vi "Verzoegerung.vi"(7 "Abfallverzögerung?":bool, 8 "ms":u16, 9 "sec":u16, 10 "min":u16, 11 "Startsignal":bool) -> (0 "Aktuelle Zeit [sec]":sgl, 3 "Zeit abgelaufen?":bool)   [LabVIEW 2020, in "Allgemein.lvlib"]
uses:
  Allgemein.lvlib
panel:
  # "VI Einstellung:\nAblaufinvarinate Ausführung\nKopie für jede Instanz vorbelegen\n(behält Zustand für jede Instanz bei)"
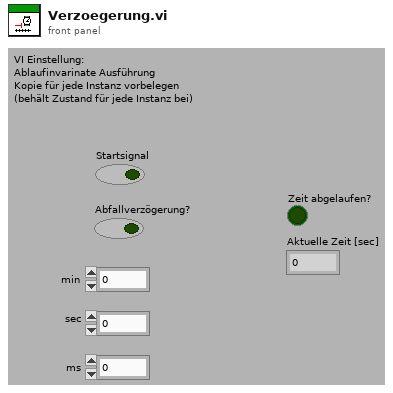
[diagram p1: front panel]
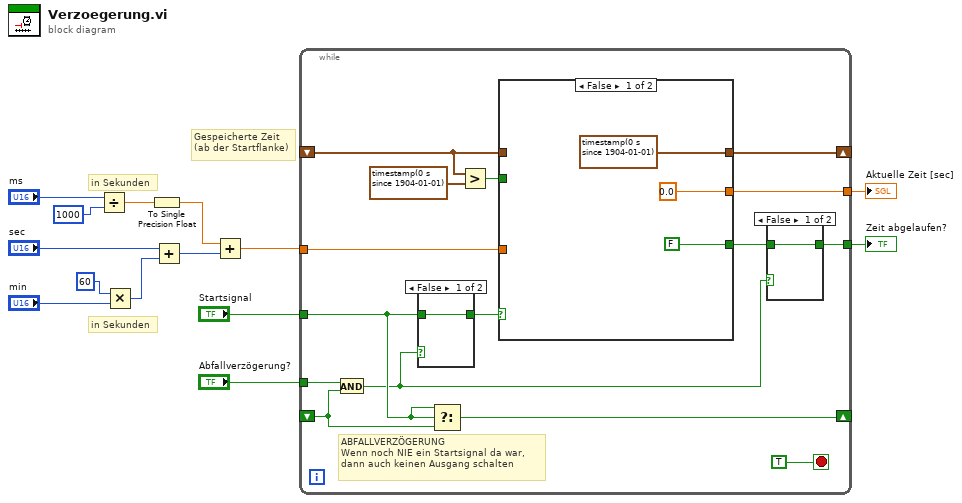
[diagram p0: block diagram]
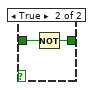
[diagram p2: hidden frame]
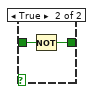
[diagram p3: hidden frame]
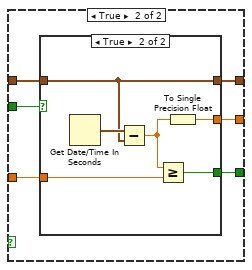
[diagram p4: hidden frame]
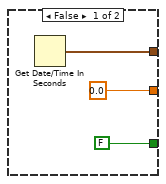
[diagram p5: hidden frame]
diagram:
  # "in Sekunden"
  # "in Sekunden"
  # "Gespeicherte Zeit\n(ab der Startflanke)"
  n1 = Divide(x="ms", y=u16 1000) -> (x/y=w3:dbl)
  n2 = Multiply(x=u16 60 ("y"), y="min") -> (x*y=w10:u16)
  n3 = To Single Precision Float(number=w3) -> (single precision float=w2:sgl)
  n4 = Add(x="sec", y=w10) -> (x+y=w6:u16)
  n5 = Add(x=w2, y=w6) -> (x+y=w5:sgl)
  n6 = while {
    shift-right: [w28] -> _
    shift-left: _ -> [w27]
    tunnel: w5 -> [w25]
    tunnel: "Startsignal" -> [w19]
    tunnel: [w24] -> w13
    tunnel: "Abfallverzögerung?" -> [w17]
    tunnel: [w20] -> w1
    shift-right: [w18] -> _
    shift-left: _ -> [w16]
    stop <- TRUE stop-if-true
    # "ABFALLVERZÖGERUNG\nWenn noch NIE ein Startsignal da war, \ndann auch keinen Ausgang schalten"
    n7 = And(x=w17, y=w16) -> (x .and. y?=w15:bool)
    n8 = case shown="False" w15 {
      tunnel: w19 -> [w33 w35]
      tunnel: [w33 w34] -> w21
      frame False {
      }
      frame True {
        n9 = Not(x=w35) -> (.not. x?=w34:bool)
      }
    }
    n10 = Select(t=w19, s=w19, f=w16) -> (s? t:f=w18:bool)
    n11 = Greater?(x=w27, y=timestamp(0 s since 1904-01-01) ("Aktuelle Zeit")) -> (0:w26:bool)
    n12 = case shown="False" w21 {
      tunnel: [timestamp(0 s since 1904-01-01) ("Aktuelle Zeit") w44] -> w28
      tunnel: w27 -> [_ w42]
      tunnel: w26 -> [_ w43]
      tunnel: w25 -> [_ w41]
      tunnel: [FALSE w40] -> w22
      tunnel: [sgl 0.0 w39] -> w24
      frame False {
      }
      frame True {
        n13 = case shown="True" w43 {
          tunnel: [w47 w51] -> w44
          tunnel: w42 -> [_ w51]
          tunnel: w41 -> [_ w52]
          tunnel: [FALSE w50] -> w40
          tunnel: [sgl 0.0 w49] -> w39
          frame False {
            n14 = Get Date/Time In Seconds() -> (seconds since 1Jan1904=w47:timestamp)
          }
          frame True {
            n15 = Get Date/Time In Seconds() -> (seconds since 1Jan1904=w53:timestamp)
            n16 = Subtract(x=w53, y=w51) -> (x-y=w48:dbl)
            n17 = Greater Or Equal?(x=w48, y=w52) -> (x >= y?=w50:bool)
            n18 = To Single Precision Float(number=w48) -> (single precision float=w49:sgl)
          }
        }
      }
    }
    n19 = case shown="False" w15 {
      tunnel: w22 -> [w30 w32]
      tunnel: [w30 w31] -> w20
      frame False {
      }
      frame True {
        n20 = Not(x=w32) -> (.not. x?=w31:bool)
      }
    }
  }
  "Zeit abgelaufen?" <- w1
  "Aktuelle Zeit [sec]" <- w13
